vi "CS POLARIS BME DG.Create DIMServices.vi"(8 "error in (no error)":errorcluster, 10 "objname":string, 11 "BME_DG_System in":refnum<class "BME_DG_System.lvclass">) -> (0 "error out":errorcluster, 3 "BME_DG_System out":refnum<class "BME_DG_System.lvclass">)   [LabVIEW 2009, in "CS POLARIS BME DG.lvlib"]
uses:
  CS POLARIS BME DG.lvlib
  DG Classes/BME_DG_System/BME_DG_System.lvclass
  DG Classes/BME_DG_Base/BME_DG_Base.lvclass
  DG Classes/BME_DG_Chnl/BME_DG_Chnl.lvclass
  lib.lib/DimLVEvent/LVDimInterface/LVDimInterface.lvlib
panel:
  in  "typeDescriptor":string
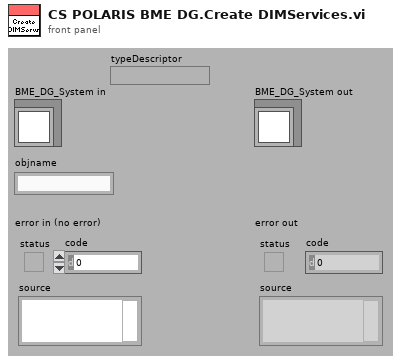
[diagram p1: front panel]
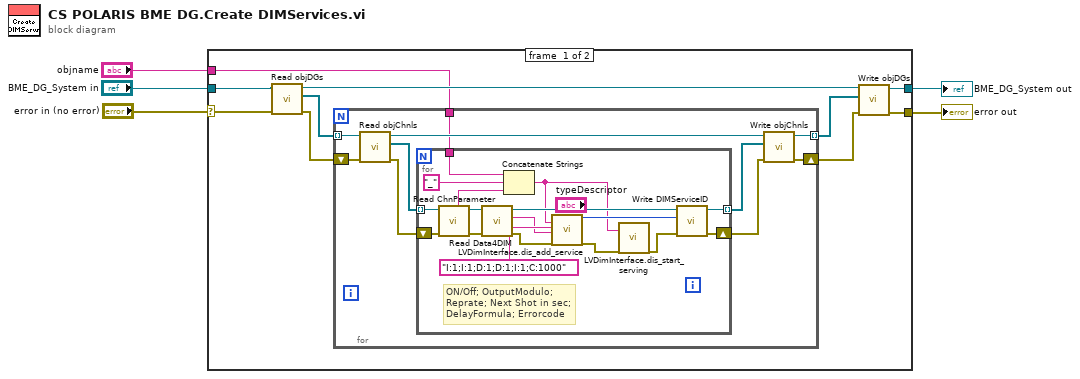
[diagram p0: block diagram]
diagram:
  n1 = case shown="No Error" "error in (no error)" {
    selector: "error in (no error)" -> [w14 w44]
    tunnel: [w6 w44] -> w4
    tunnel: "BME_DG_System in" -> [w15 w43]
    tunnel: [w11 w43] -> w2
    tunnel: "objname" -> [w8 _]
    frame #0 {
      n2 = call "Read objDGs.vi"("error in (no error)"=w14, "BME_DG_System in"=w15) -> ("error out"=w9:errorcluster, "objDGs"=w13:refnum<class "BME_DG_Base.lvclass">[], "BME_DG_System out"=w12:refnum<class "BME_DG_System.lvclass">)  [unwired: 7 in]
      n3 = for {
        tunnel: w13 -> [w25] mode=indexing
        tunnel: [w23] -> w10 mode=indexing
        shift-right: [w19] -> w7
        shift-left: w9 -> [w18]
        tunnel: w8 -> [w17]
        n4 = call-dynamic "Read objChnls.vi"("error in (no error)"=w18, "BME_DG_Base in"=w25) -> ("error out"=w21:errorcluster, "objChnls"=w22:refnum<class "BME_DG_Chnl.lvclass">[], "BME_DG_Base out"=w24:refnum<class "BME_DG_Base.lvclass">)  [unwired: 6 in, 1 out]
        n5 = for {
          tunnel: w22 -> [w41] mode=indexing
          tunnel: [w40] -> w20 mode=indexing
          shift-right: [w39] -> w16
          shift-left: w21 -> [w42]
          tunnel: w17 -> [w37]
          # "ON/Off; OutputModulo;\nReprate; Next Shot in sec;\nDelayFormula; Errorcode"
          n6 = call-dynamic "Read ChnParameter.vi"("error in (no error)"=w42, "BME_DG_Chnl in"=w41) -> ("error out"=w33:errorcluster, "BME_DG_Chnl out"=w32:refnum<class "BME_DG_Chnl.lvclass">, "Name"=w35:string)  [unwired: 4 in, 3 out]
          n7 = call-dynamic "Read Data4DIM.vi"("error in (no error)"=w33, "BME_DG_Chnl in"=w32) -> ("error out"=w30:errorcluster, "DIMData"=w29:string, "BME_DG_Chnl out"=w31:refnum<class "BME_DG_Chnl.lvclass">)  [unwired: 6 in, 1 out]
          n8 = Concatenate Strings(w37, "_" ("string"), w35) -> (w27:string)
          n9 = call "LVDimInterface.dis_add_service.vi"("serviceName"=w27, "typeDescriptor"="I:1;I:1;D:1;D:1;I:1;C:1000", "data"=w29, "error in (no error)"=w30) -> ("my_serviceID"=w38:i32, "error out"=w28:errorcluster)  [unwired: 14 in]
          n10 = call "LVDimInterface.dis_start_serving.vi"("serverName"=w27, "error in (no error)"=w28) -> ("error out"=w26:errorcluster)  [unwired: 16 in, 1 out]
          n11 = call-dynamic "Write DIMServiceID.vi"("error in (no error)"=w26, "DIMServiceID"=w38, "BME_DG_Chnl in"=w31) -> ("error out"=w39:errorcluster, "BME_DG_Chnl out"=w40:refnum<class "BME_DG_Chnl.lvclass">)  [unwired: 7 in]
        }
        n12 = call-dynamic "Write objChnls.vi"("error in (no error)"=w16, "objChnls"=w20, "BME_DG_Base in"=w24) -> ("error out"=w19:errorcluster, "BME_DG_Base out"=w23:refnum<class "BME_DG_Base.lvclass">)  [unwired: 7 in]
      }
      n13 = call "Write objDGs.vi"("error in (no error)"=w7, "objDGs"=w10, "BME_DG_System in"=w12) -> ("error out"=w6:errorcluster, "BME_DG_System out"=w11:refnum<class "BME_DG_System.lvclass">)  [unwired: 7 in]
    }
    frame #1 {
    }
  }
  "error out" <- w4
  "BME_DG_System out" <- w2
